vi "Up Down Hall.vi"() -> ()   [LabVIEW 2021]
uses:
  6c21c491-3613-49b9-8739-58848ace7e6b.vi
  9d677228-37d7-4fae-91d8-cc659d765936.vi
  9a2c7101-15d1-4822-83f9-fc476c468639.vi
  af5d74b8-55dd-445e-b05f-4c49f1f30415.vi
panel:
  in  "Stop":bool
  in  "Save":bool
  in  "Configuration":T1={"Up file"=path "", "Down file"=path "", "Invert X"=TRUE, "Bin data"=enum."Down", "Bin size"=0.1, "Chan Vxy X"="V X1 (Resampled)", "Chan Vxy Y"="V Y1 (Resampled)", "Chan X"="Field (Resampled)", "Group"="p", "Phase"=0.0, "Delta Phase"=0.0, "Averaging"=0.0, "Output file name"="Hall_100K"} {"Delta Phase" step=0.05 scale=-180.0..180.0; "Phase" scale=-180.0..180.0}
  out "Hall":T2(graph)
  out "Vxy":T2(graph)
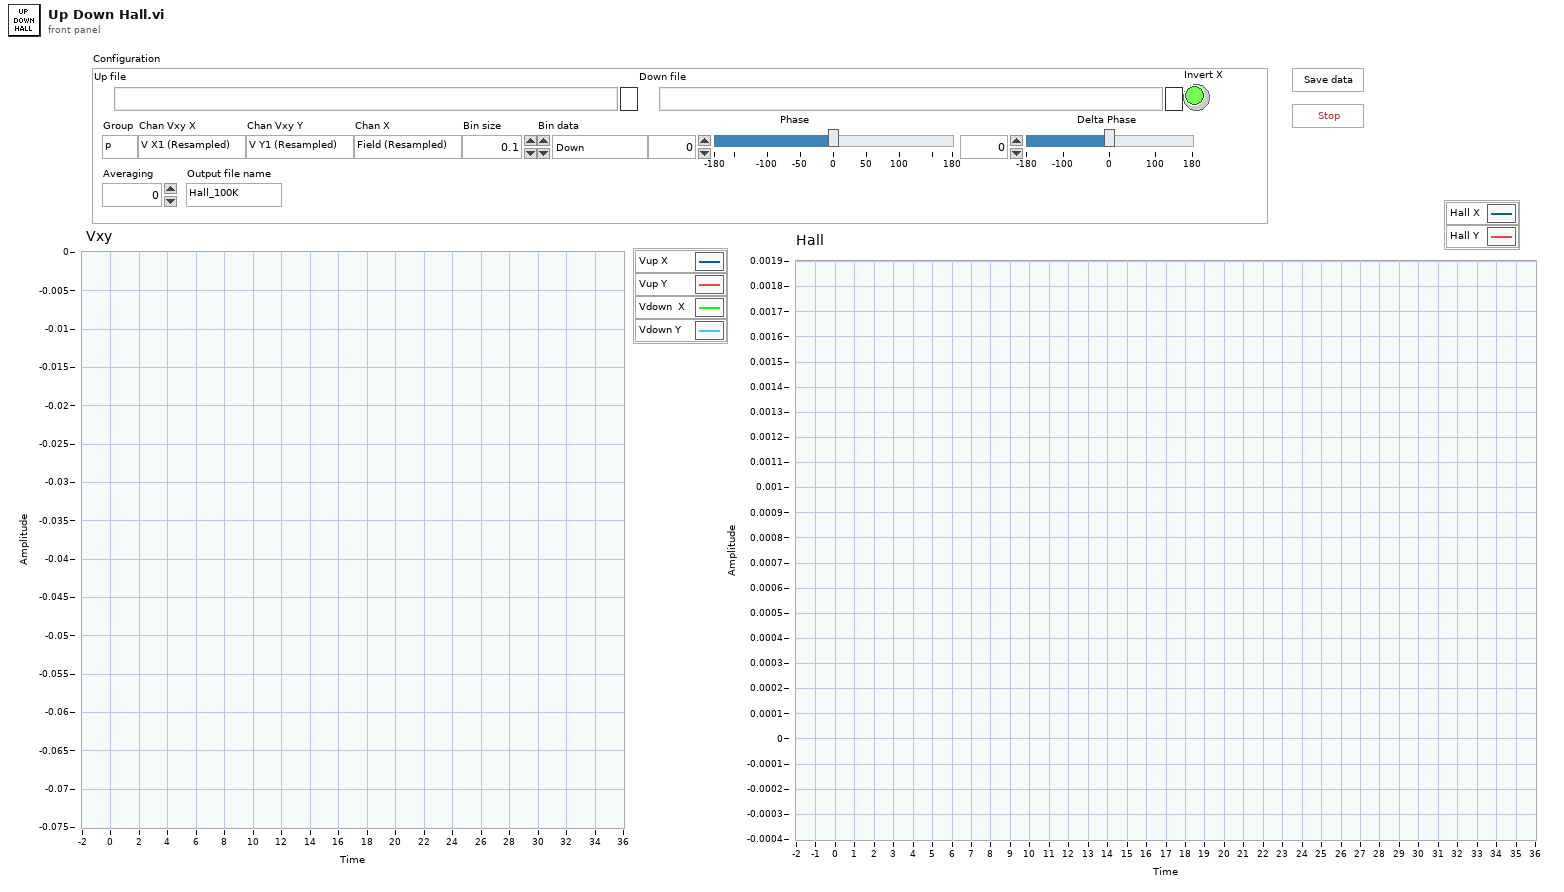
[diagram p1: front panel]
types:
  T1 = cluster{"Up file":path, "Down file":path, "Invert X":bool, "Bin data":enum16{"NONE", "Up", "Down", "Up+Down"}, "Bin size":dbl, "Chan Vxy X":string, "Chan Vxy Y":string, "Chan X":string, "Group":string, "Phase":dbl, "Delta Phase":dbl, "Averaging":dbl, "Output file name":string}
  T2 = cluster{"Binned data up":dbl[], "Binned data up":dbl[]}[]
  T3 = enum16{"open", "open or create", "create or replace", "create", "open (read-only)"}
  T4 = cluster{"Binned data down":dbl[], "Array X out":dbl[]}
  T5 = cluster{"Binned data down":dbl[], "Array Y out":dbl[]}
  T6 = cluster{"Binned data down":dbl[], "Array Y out":dbl[]}[]
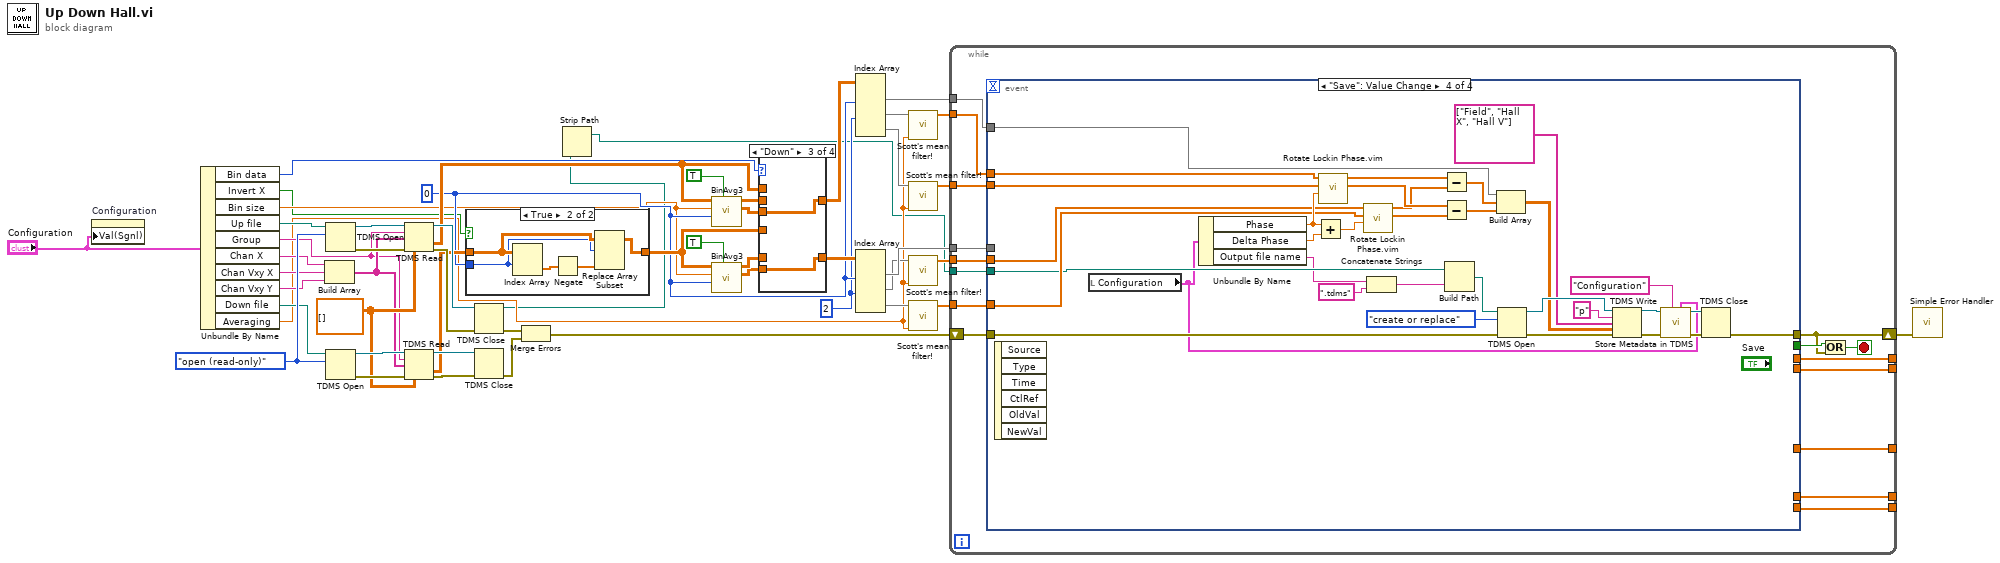
[diagram p0: block diagram]
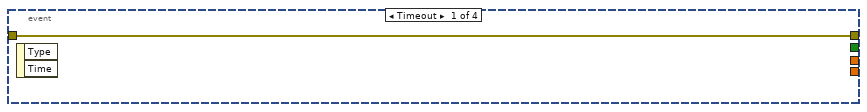
[diagram p3: hidden frame]
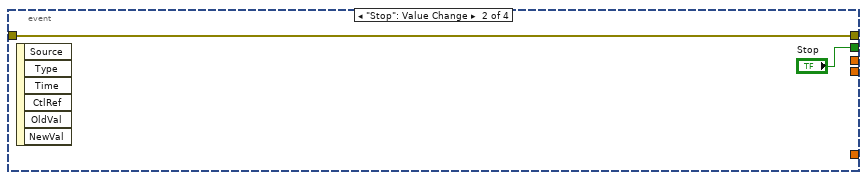
[diagram p4: hidden frame]
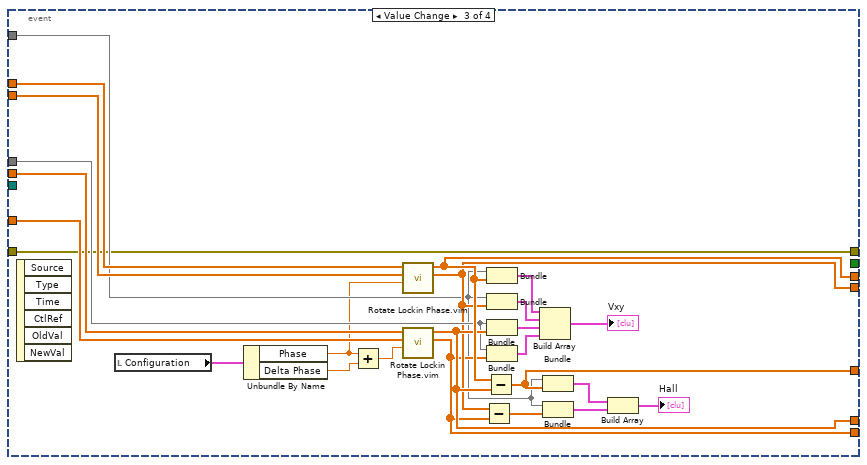
[diagram p5: hidden frame]
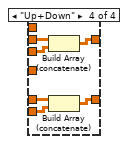
[diagram p8: hidden frame]
diagram:
  w20 = 2 ("index (row)")
  w21 = 0 ("index (row)")
  w42 = dbl[][] []
  w43 = T3."open (read-only)" ("operation (0:open)")
  n1 = property on="Configuration" class="Clust (strict)"("Val(Sgnl)"="Configuration") -> ()  [unwired: 2 in, 2 out]
  n2 = Unbundle By Name("Configuration") -> ("Bin data"=w8:enum16{"NONE", "Up", "Down", "Up+Down"}, "Invert X"=w7:bool, "Bin size"=w11:dbl, "Up file"=w19:path, "Group"=w15:string, "Chan X"=w16:string, "Chan Vxy X"=w18:string, "Chan Vxy Y"=w17:string, "Down file"=w14:path, "Averaging"=w10:dbl)
  n3 = Build Array(w16, w18, w17) -> (w41:string[])
  n4 = TDMS Open(10:w43, 11:w19) -> (0:w50:errorcluster, 3:w51:refnum<k34>)  [unwired: 5 in]
  n5 = TDMS Open(10:w43, 11:w14) -> (0:w45:errorcluster, 3:w44:refnum<k34>)  [unwired: 5 in]
  n6 = TDMS Read(0:w51, 5:w15, 7:w41, 11:w50, 12:w42) -> (4:w48:refnum<k34>, 10:w38:dbl[][], 15:w49:errorcluster)  [unwired: 3 in, 3 out]
  n7 = TDMS Read(0:w44, 5:w15, 7:w41, 11:w45, 12:w42) -> (4:w47:refnum<k34>, 10:w23:dbl[][], 15:w46:errorcluster)  [unwired: 3 in, 3 out]
  n8 = case shown="True" w7 {
    tunnel: w23 -> [w52 w57]
    tunnel: w21 -> [_ w54]
    tunnel: [w52 w53] -> w22
    frame False {
    }
    frame True {
      n9 = Index Array(array=w57, index (row)=w54) -> (element=w56:dbl[])  [unwired: 1 in]
      n10 = Negate(x=w56) -> (-x=w55:dbl[])
      n11 = Replace Array Subset(array=w57, new element=w55, index (row)=w54) -> (w53:dbl[][])  [unwired: 1 in]
    }
  }
  n12 = TDMS Close(8:w49, 11:w48) -> (0:w3:errorcluster, 3:w6:path)
  n13 = TDMS Close(8:w46, 11:w47) -> (0:w4:errorcluster)  [unwired: 1 out]
  n14 = Merge Errors(w3, w4) -> (w2:errorcluster)
  n15 = Strip Path(path=w6) -> (stripped path=w5:path)  [unwired: 1 out]
  n16 = call "BinAvg3.vi"("Extend to 0"=TRUE, "X coumn index"=w21, "Bin size"=w11, "Data in"=w38) -> ("Binned data down"=w36:dbl[][], "Binned data up"=w39:dbl[][])  [unwired: 6 in]
  n17 = call "BinAvg3.vi"("Extend to 0"=TRUE, "X coumn index"=w21, "Bin size"=w11, "Data in"=w22) -> ("Binned data down"=w37:dbl[][], "Binned data up"=w40:dbl[][])  [unwired: 6 in]
  n18 = case shown="\"Down\"" w8 {
    tunnel: w40 -> [_ w61 _ w69]
    tunnel: [w59 w61 w63 w67] -> w29
    tunnel: w39 -> [_ w60 _ w66]
    tunnel: [w58 w60 w62 w64] -> w35
    tunnel: w22 -> [w59 _ _ _]
    tunnel: w38 -> [w58 _ _ _]
    tunnel: w37 -> [_ _ w63 w68]
    tunnel: w36 -> [_ _ w62 w65]
    frame "NONE", Default {
    }
    frame "Up" {
    }
    frame "Down" {
    }
    frame "Up+Down" {
      n19 = Build Array (concatenate)(w66, w65) -> (w64:dbl[][])
      n20 = Build Array (concatenate)(w69, w68) -> (w67:dbl[][])
    }
  }
  n21 = Index Array(array=w35, index (col) #1=w21, index (col) #2=w20) -> (element #1=w34:dbl[], element #2=w25:dbl[], element #3=w24:dbl[])  [unwired: 4 in]
  n22 = Index Array(array=w29, index (col) #1=w21, index (col) #2=w20) -> (element #1=w28:dbl[], element #2=w27:dbl[], element #3=w26:dbl[])  [unwired: 4 in]
  n23 = call "Scott's mean filter!.vi"("window size"=w10, "input"=w25) -> ("output"=w33:dbl[])  [unwired: 9 out]
  n24 = call "Scott's mean filter!.vi"("window size"=w10, "input"=w24) -> ("output"=w32:dbl[])  [unwired: 9 out]
  n25 = call "Scott's mean filter!.vi"("window size"=w10, "input"=w27) -> ("output"=w31:dbl[])  [unwired: 9 out]
  n26 = call "Scott's mean filter!.vi"("window size"=w10, "input"=w26) -> ("output"=w30:dbl[])  [unwired: 9 out]
  n27 = while {
    tunnel: [w78] -> _
    tunnel: [w80] -> _
    tunnel: [w77] -> _
    tunnel: [w81] -> _
    tunnel: [w79] -> _
    tunnel: w30 -> [w82]
    tunnel: w31 -> [w83]
    tunnel: w32 -> [w84]
    tunnel: w33 -> [w85]
    tunnel: w34 -> [w75]
    tunnel: w28 -> [w74]
    tunnel: w5 -> [w73]
    shift-right: [w71] -> w1
    shift-left: w2 -> [w70]
    stop <- w72 stop-if-true
    n28 = event shown="[3] \"Save\": Value Change" {
      selector: _ -> [_ _ _ _]
      dyn-events: _ -> [_ _ _ _]
      timeout: _ -> [_ _ _ _]
      tunnel: w85 -> [_ _ w113 w136]
      tunnel: w84 -> [_ _ w112 w135]
      tunnel: w83 -> [_ _ w111 w134]
      tunnel: w82 -> [_ _ w110 w133]
      tunnel: [_ _ w101 _] -> w81
      tunnel: [_ _ w100 _] -> w80
      tunnel: [_ _ w109 _] -> w79
      tunnel: [_ _ w99 _] -> w78
      tunnel: [_ _ w105 _] -> w77
      tunnel: [_ "Stop" _ _] -> w76
      tunnel: w75 -> [_ _ w97 w140]
      tunnel: w74 -> [_ _ w104 _]
      tunnel: w73 -> [_ _ _ w132]
      tunnel: w70 -> [w86 w87 w89 w128]
      tunnel: [w86 w87 w89 w123] -> w71
      event Timeout {
        n29 = event-data() -> ()  [unwired: 3 out]
      }
      event "Stop": Value Change {
        n30 = event-data() -> ()  [unwired: 7 out]
      }
      event "Configuration.Phase", "Configuration.Delta Phase": Value Change {
        n31 = event-data() -> ()  [unwired: 7 out]
        n32 = local read "Configuration"() -> (w92:T1)
        n33 = Unbundle By Name(w92) -> ("Phase"=w91:dbl, "Delta Phase"=w90:dbl)
        n34 = Add(x=w91, y=w90) -> (x+y=w93:dbl)
        n35 = call "Rotate Lockin Phase.vim"("Phase"=w91, "Array Y in"=w112, "Array X in"=w113) -> ("Array Y out"=w101:dbl[], "Array X out"=w109:dbl[])  [unwired: 7 in]
        n36 = call "Rotate Lockin Phase.vim"("Phase"=w93, "Array Y in"=w110, "Array X in"=w111) -> ("Array Y out"=w100:dbl[], "Array X out"=w105:dbl[])  [unwired: 7 in]
        n37 = Subtract(x=w101, y=w100) -> (x-y=w98:dbl[])
        n38 = Subtract(x=w109, y=w105) -> (x-y=w99:dbl[])
        n39 = Bundle("Binned data down"=w97, "Array X out"=w109) -> (w108:T4)  [unwired: 1 in]
        n40 = Bundle("Binned data down"=w97, "Array Y out"=w101) -> (w107:T5)  [unwired: 1 in]
        n41 = Bundle("Binned data down"=w104, "Array X out"=w105) -> (w102:T4)  [unwired: 1 in]
        n42 = Bundle("Binned data down"=w104, "Array Y out"=w100) -> (w103:T5)  [unwired: 1 in]
        n43 = Build Array(w108, w107, w102, w103) -> (→"Vxy":T6)
        n44 = Bundle("Binned data down"=w97, w99) -> (w96:cluster{"Binned data down":dbl[], dbl[]})  [unwired: 1 in]
        n45 = Bundle("Binned data down"=w97, w98) -> (w95:cluster{"Binned data down":dbl[], dbl[]})  [unwired: 1 in]
        n46 = Build Array(w96, w95) -> (→"Hall":cluster{"Binned data down":dbl[], dbl[]}[])
      }
      event "Save": Value Change {
        n47 = event-data() -> ()  [unwired: 7 out]
        n48 = local read "Configuration"() -> (w115:T1)
        n49 = Unbundle By Name(w115) -> ("Phase"=w142:dbl, "Delta Phase"=w141:dbl, "Output file name"=w131:string)
        n50 = Add(x=w142, y=w141) -> (x+y=w143:dbl)
        n51 = call "Rotate Lockin Phase.vim"("Phase"=w142, "Array Y in"=w135, "Array X in"=w136) -> ("Array Y out"=w145:dbl[], "Array X out"=w146:dbl[])  [unwired: 7 in]
        n52 = call "Rotate Lockin Phase.vim"("Phase"=w143, "Array Y in"=w133, "Array X in"=w134) -> ("Array Y out"=w144:dbl[], "Array X out"=w137:dbl[])  [unwired: 7 in]
        n53 = Concatenate Strings(w131, ".tdms") -> (w129:string)
        n54 = Subtract(x=w146, y=w137) -> (x-y=w139:dbl[])
        n55 = Subtract(x=w145, y=w144) -> (x-y=w138:dbl[])
        n56 = Build Path(base path=w132, name or relative path=w129) -> (appended path=w127:path)
        n57 = Build Array(w140, w139, w138) -> (w120:dbl[][])
        n58 = TDMS Open(8:w128, 10:T3."create or replace" ("operation (0:open)"), 11:w127) -> (0:w125:errorcluster, 3:w124:refnum<k34>)  [unwired: 4 in]
        n59 = TDMS Write(0:w124, 5:"p" ("group name in (Untitled)"), 7:string[] ["Field", "Hall X", "Hall V"] ("channel name(s) in (Untitled)"), 9:w120, 11:w125) -> (4:w119:refnum<k34>, 15:w116:errorcluster)  [unwired: 1 in, 2 out]
        n60 = call "Store Metadata in TDMS.vi"("Value"=w115, "name"="Configuration", "Error In"=w116, "tdms file"=w119) -> ("Error Out"=w117:errorcluster, "tdms file out"=w118:refnum<k34>)  [unwired: 3 in, 3 out]
        n61 = TDMS Close(8:w117, 11:w118) -> (0:w123:errorcluster)  [unwired: 1 out]
      }
    }
    n62 = Or(x=w76, y=w71) -> (x .or. y?=w72:bool)
  }
  n63 = call <vilib>:"Simple Error Handler.vi"("error in (no error)"=w1) -> ()  [unwired: 4 in, 5 out]
